vi "Cobra_Front_Panel_Vision_4k.vi"() -> ()   [LabVIEW 2015]
uses:
  <vilib>/vision/Measure.llb/Edge Options.ctl
  <vilib>/vision/Measure.llb/Edge Polarity.ctl
  <vilib>/vision/NI_Vision_Development_Module.lvlib
panel:
  in  "Save Button":bool
  in  "RESET Button":bool
  in  "Process":T1(ring)=enum."Get All Edges"
  in  "Edge Options":T2={"Edge Polarity"=0, "Kernel Size"=3, "Width"=3, "Minimum Edge Strength"=10.0, "Interpolation Type"=enum."Bilinear Fixed", "Data Processing Method"=enum."Average"} {"Edge Polarity" items=["All Edges", "Rising Edges", "Falling Edges"]; "Minimum Edge Strength" format="%.2f"; "Width" step=2; "Kernel Size" step=2}
  out "Line Profile":cluster{"x0":sgl, "dx":sgl, "Pixels Line":sgl[]}(graph)={"x0"=0.0, "dx"=1.0, "Pixels Line"=[]}
  out "Image":T4(plugin-control)
  out "Gradient Information":dbl[](graph)
  in  "Internal Trigger":bool=TRUE
  in  "EXIT":bool
  in  "Line Scan Enable":bool=TRUE
  in  "Line Time Value":u16=90 step=1
  in  "Integration Time Value":u16=100 min=1 max=32767 step=1
  in  "Offset Value":u16=255 max=255 step=1
  in  "Gain Value":u16=187 max=255 step=1
  out "Configuration String Sent":string
  out "Failure":bool
  out "Initialized":bool
  in  "Set":bool
  out "Characters Read":u32
  out "IMAQ Session Out":refnum<k11>
  out "Command Data Read":string
  out "Error Output":errorcluster
  in  "error in (no error)":errorcluster
  # "Suggested Starting Values:\n\nGain: 187\nOffset: 255\nIntegration Time: 90\nLine Time: 100"
  # "Inital Setup and Connection:\n\n  1. Launch NI MAX, select the camera (should be img0).\n  2. Load the supplied *.icd file for the camera.\n  3. Close NI MAX.\n  4. Run this VI and click the \"Set all\" button.\n  5. Stop VI, wait two seconds and run it again to view data"
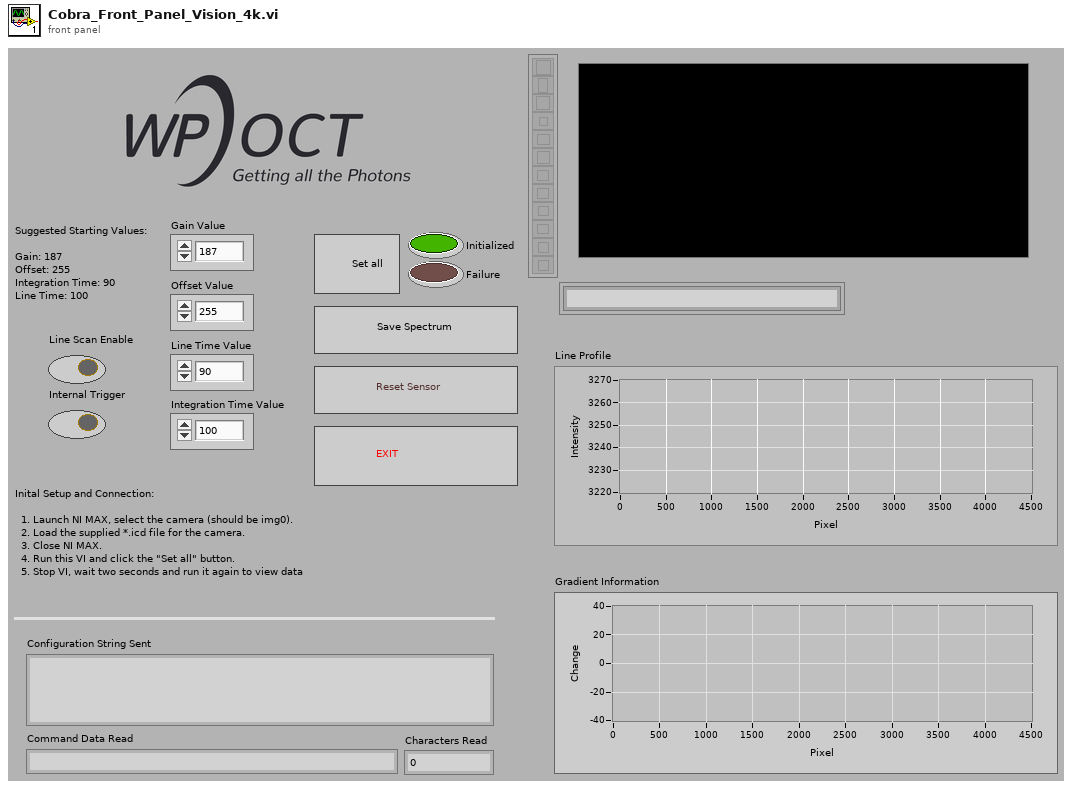
[diagram p1: front panel]
types:
  T1 = enum16{"Get First Edge", "Get First + Last Edge", "Get All Edges", "Get Best Edge"}
  T2 = typedef "Edge Options.ctl" = cluster{"Edge Polarity":T3, "Kernel Size":u32, "Width":u32, "Minimum Edge Strength":sgl, "Interpolation Type":enum32{"Zero Order", "Bilinear", "Quadratic", "Cubic", "Bilinear Fixed"}, "Data Processing Method":enum32{"Average", "Median"}}
  T3 = typedef "Edge Polarity.ctl" = u32
  T4 = typedef "IMAQ Image.ctl" = refnum<image>
  T5 = cluster{"Global Rectangle":i32[], "Contours":cluster{"Contour Type":u32, "ROI Type":u32, "Points":i32[]}[]}
  T6 = typedef "Edge New.ctl" = cluster{"Location (Pixel)":cluster{"X":sgl, "Y":sgl}, "Location (Real-World)":cluster{"X":sgl, "Y":sgl}, "Distance (Pixel)":dbl, "Distance (Real-World)":dbl, "Strength":dbl, "Noise":dbl, "Rising?":bool}
  T7 = typedef "imagedata.ctl" = cluster{"image type":i32, "image depth":i32, "image":u8[], "mask":u8[], "colors":u32[], "Rectangle":cluster{"left":i16, "top":i16, "right":i16, "bottom":i16}}
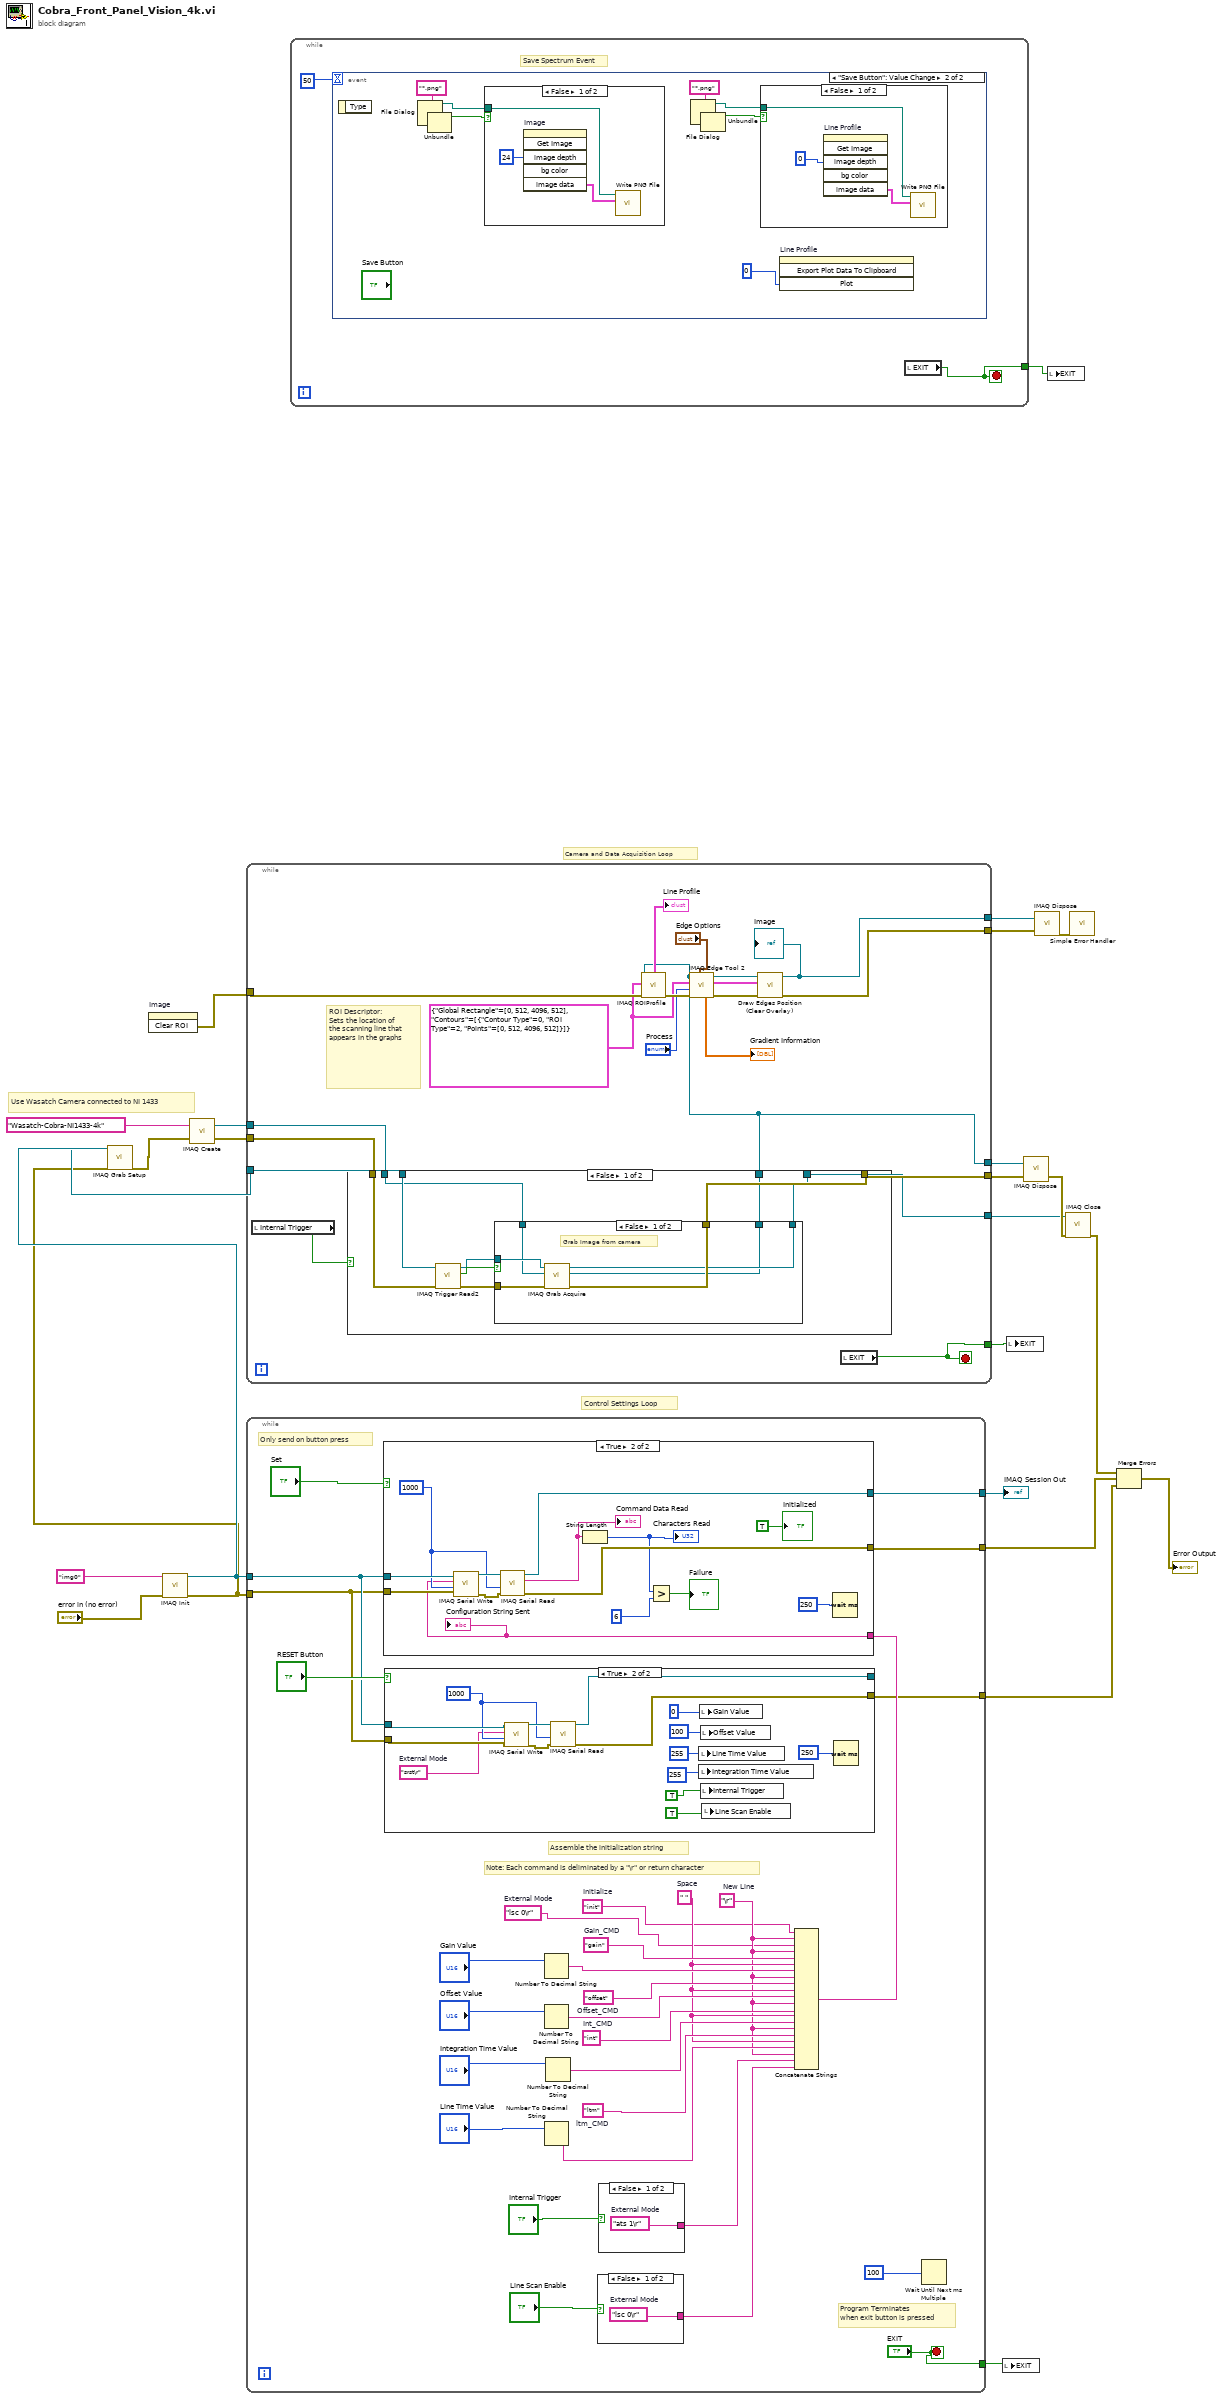
[diagram p0: block diagram]
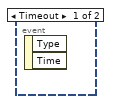
[diagram p2: hidden frame]
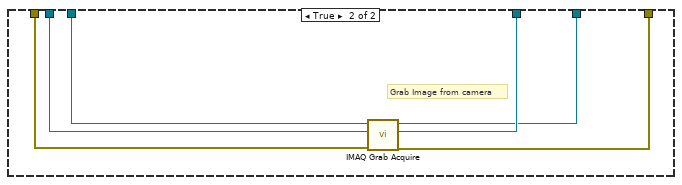
[diagram p6: hidden frame]
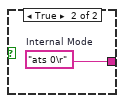
[diagram p8: hidden frame]
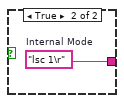
[diagram p10: hidden frame]
diagram:
  # "Use Wasatch Camera connected to NI 1433"
  # "Camera and Data Acquisition Loop"
  # "Control Settings Loop"
  n1 = invoke on="Image" class="ImageControl" method="Clear ROI"() -> (error out=w7:errorcluster)  [unwired: 3 in, 2 out]
  n2 = call <vilib>:"IMAQ Init.vi"("error in (no error)"="error in (no error)", "Interface Name"="img0") -> ("error out"=w21:errorcluster, "IMAQ Session Out"=w23:refnum<k11>)  [unwired: 8 in]
  n3 = call <vilib>:"IMAQ Grab Setup.vi"("error in (no error)"=w21, "IMAQ Session In"=w23) -> ("error out"=w20:errorcluster, "IMAQ Session Out"=w22:refnum<k11>)  [unwired: 8 in]
  n4 = call "IMAQ Create"("Image Name"="Wasatch-Cobra-NI1433-4k", "error in (no error)"=w20) -> ("New Image"=w18:T4, "error out"=w19:errorcluster)  [unwired: 3 in]
  n5 = while {
    tunnel: w23 -> [w29]
    tunnel: w21 -> [w28]
    tunnel: [w55] -> w24
    tunnel: [w54] -> w13
    tunnel: [w27] -> w4
    tunnel: ["EXIT"] -> w3
    stop <- "EXIT" stop-if-true
    w35 = "lsc 0\r"  # External Mode
    w43 = "ltm"  # ltm_CMD
    w42 = "int"  # Int_CMD
    w41 = "offset"  # Offset_CMD
    w40 = "gain"  # Gain_CMD
    w37 = " "  # Space
    w36 = "\r"  # New Line
    w34 = "init"  # Initialize
    # "Program Terminates\nwhen exit button is pressed"
    # "Only send on button press"
    # "Note: Each command is deliminated by a \"\\r\" or return character"
    # "Assemble the initialization string"
    n6 = case shown="True" "RESET Button" {
      tunnel: w29 -> [w57 w67]
      tunnel: w28 -> [w56 w65]
      tunnel: [w57 w72] -> _
      tunnel: [w56 w71] -> w27
      frame False {
      }
      frame True {
        w64 = "srst\r"  # External Mode
        w66 = 1000
        n7 = call <vilib>:"IMAQ Serial Write.vi"("error in (no error)"=w65, "Timeout"=w66, "String to write"=w64, "IMAQ Session In"=w67) -> ("error out"=w68:errorcluster, "IMAQ Session Out"=w69:refnum<k11>)  [unwired: 4 in]
        n8 = call <vilib>:"IMAQ Serial Read.vi"("error in (no error)"=w68, "Timeout"=w66, "IMAQ Session In"=w69) -> ("error out"=w71:errorcluster, "IMAQ Session Out"=w72:refnum<k11>)  [unwired: 3 in, 2 out]
        n9 = local write "Line Time Value"(255) -> ()
        n10 = local write "Integration Time Value"(255) -> ()
        n11 = local write "Gain Value"(0) -> ()
        n12 = local write "Offset Value"(100) -> ()
        n13 = local write "Internal Trigger"(TRUE) -> ()
        n14 = local write "Line Scan Enable"(TRUE) -> ()
        n15 = Wait (ms)(milliseconds to wait=250) -> ()  [unwired: 1 out]
      }
    }
    n16 = Number To Decimal String(number="Gain Value") -> (decimal integer string=w44:string)  [unwired: 1 in]
    n17 = Number To Decimal String(number="Offset Value") -> (decimal integer string=w46:string)  [unwired: 1 in]
    n18 = Number To Decimal String(number="Line Time Value") -> (decimal integer string=w51:string)  [unwired: 1 in]
    n19 = Number To Decimal String(number="Integration Time Value") -> (decimal integer string=w49:string)  [unwired: 1 in]
    n20 = case shown="False" "Line Scan Enable" {
      tunnel: [w91 w92] -> w31
      frame False {
        w91 = "lsc 0\r"  # External Mode
      }
      frame True {
        w92 = "lsc 1\r"  # Internal Mode
      }
    }
    n21 = case shown="False" "Internal Trigger" {
      tunnel: [w73 w74] -> w32
      frame False {
        w73 = "ats 1\r"  # External Mode
      }
      frame True {
        w74 = "ats 0\r"  # Internal Mode
      }
    }
    n22 = Concatenate Strings(w34, w36, w35, w36, w40, w37, w44, w36, w41, w37, w46, w36, w42, w37, w49, w36, w43, w37, w51, w36, w32, w31) -> (w39:string)
    n23 = case shown="True" "Set" {
      tunnel: w29 -> [w76 w84]
      tunnel: w28 -> [w75 w82]
      tunnel: [w76 w90] -> w55
      tunnel: [w75 w89] -> w54
      tunnel: w39 -> [_ w81]
      frame False {
      }
      frame True {
        w83 = 1000
        n24 = call <vilib>:"IMAQ Serial Write.vi"("error in (no error)"=w82, "Timeout"=w83, "String to write"=w81, "IMAQ Session In"=w84) -> ("error out"=w85:errorcluster, "IMAQ Session Out"=w86:refnum<k11>)  [unwired: 4 in]
        n25 = call <vilib>:"IMAQ Serial Read.vi"("error in (no error)"=w85, "Timeout"=w83, "IMAQ Session In"=w86) -> ("error out"=w89:errorcluster, "String Read"=w80:string, "IMAQ Session Out"=w90:refnum<k11>)  [unwired: 3 in, 1 out]
        "Command Data Read" <- w80
        n26 = String Length(string=w80) -> (length=w79:i32)
        "Characters Read" <- w79
        n27 = Greater?(x=w79, y=6) -> (0:→"Failure":bool)
        n28 = Wait (ms)(milliseconds to wait=250) -> ()  [unwired: 1 out]
        "Configuration String Sent" <- w81
        "Initialized" <- TRUE
      }
    }
    n29 = Wait Until Next ms Multiple(millisecond multiple=100) -> ()  [unwired: 1 out]
  }
  "IMAQ Session Out" <- w24
  n30 = while {
    tunnel: w22 -> [w97]
    tunnel: w19 -> [w99]
    tunnel: w18 -> [w98]
    tunnel: [w96] -> w17
    tunnel: [w95] -> w16
    tunnel: [w94] -> w14
    tunnel: w7 -> [w106]
    tunnel: [w105] -> w6
    tunnel: [w102] -> w5
    tunnel: [w101] -> w2
    stop <- w101 stop-if-true
    w93 = T5 {"Global Rectangle"=[0, 512, 4096, 512], "Contours"=[{"Contour Type"=0, "ROI Type"=2, "Points"=[0, 512, 4096, 512]}]} ("NewVal")
    # "ROI Descriptor:\nSets the location of the scanning line that appears in the graphs"
    n31 = local read "Internal Trigger"() -> (w100:bool)
    n32 = case shown="False" w100 {
      tunnel: w99 -> [w119 w135]
      tunnel: w98 -> [w115 w134]
      tunnel: w97 -> [w120 w133]
      tunnel: [w114 w132] -> w96
      tunnel: [w112 w131] -> w95
      tunnel: [w113 w130] -> w94
      frame False {
        n33 = call <vilib>:"IMAQ Trigger Read2.vi"("error in (no error)"=w119, "IMAQ Session In"=w120) -> ("error out"=w118:errorcluster, "Trigger status"=w117:bool, "IMAQ Session Out"=w116:refnum<k11>)  [unwired: 7 in]
        n34 = case shown="False" w117 {
          tunnel: w118 -> [w126 w129]
          tunnel: w116 -> [w125 w128]
          tunnel: w115 -> [w124 w127]
          tunnel: [w123 w129] -> w114
          tunnel: [w122 w128] -> w113
          tunnel: [w121 w127] -> w112
          frame False {
            # "Grab Image from camera"
            n35 = call <vilib>:"IMAQ Grab Acquire.vi"("error in (no error)"=w126, "Image In"=w124, "IMAQ Session In"=w125) -> ("error out"=w123:errorcluster, "Image Out"=w121:T4, "IMAQ Session Out"=w122:refnum<k11>)  [unwired: 5 in, 1 out]
          }
          frame True {
          }
        }
      }
      frame True {
        # "Grab Image from camera"
        n36 = call <vilib>:"IMAQ Grab Acquire.vi"("error in (no error)"=w135, "Image In"=w134, "IMAQ Session In"=w133) -> ("error out"=w132:errorcluster, "Image Out"=w131:T4, "IMAQ Session Out"=w130:refnum<k11>)  [unwired: 5 in, 1 out]
      }
    }
    n37 = call "IMAQ ROIProfile"("error in (no error)"=w106, "ROI Descriptor"=w93, "Image"=w95) -> ("error out"=w111:errorcluster, "ROI Graph"=→"Line Profile":cluster{"x0":sgl, "dx":sgl, "Pixels Line":sgl[]})  [unwired: 4 out]
    n38 = call "IMAQ Edge Tool 2"("Edge Options"="Edge Options", "error in (no error)"=w111, "Process"="Process", "ROI Descriptor"=w93, "Image"=w95) -> ("error out"=w105:errorcluster, "Edge Information"=w108:T6[], "Image (duplicate)"=w109:T4, "Gradient Values"=→"Gradient Information":dbl[])  [unwired: 1 in, 2 out]
    n39 = call "Draw Edges Position (Clear Overlay).vi"("Edge Coordinates"=w108, "Source Image"=w109) -> ("Image Out"=w102:T4)  [unwired: 9 out]
    "Image" <- w102
    n40 = local read "EXIT"() -> (w101:bool)
  }
  n41 = while {
    tunnel: [w137] -> w1
    stop <- w137 stop-if-true
    # "Save Spectrum Event"
    n42 = event shown="[1] \"Save Button\": Value Change" {
      selector: _ -> [_ _]
      dyn-events: _ -> [_ _]
      timeout: 50 -> [_ _]
      event Timeout {
        n43 = event-data() -> ()  [unwired: 1 in, 2 out]
      }
      event "Save Button": Value Change {
        n44 = event-data() -> ()  [unwired: 1 in, 1 out]
        n45 = File Dialog(6:"*.png" ("pattern")) -> (0:w146:errorcluster, 1:w144:bool, 3:w143:path)  [unwired: 6 in, 1 out]
        n46 = Unbundle(w146) -> ()  [unwired: 3 out]
        n47 = case shown="False" w144 {
          tunnel: w143 -> [w152 _]
          frame False {
            n48 = invoke on="Image" class="ImageControl" method="Get Image"("image depth"=24) -> ("image data"=w150:T7)  [unwired: 5 in, 5 out]
            n49 = call <vilib>:"Write PNG File.vi"("image data"=w150, "path to PNG file"=w152) -> ()  [unwired: 8 in, 2 out]
          }
          frame True {
          }
        }
        n50 = File Dialog(6:"*.png" ("pattern")) -> (0:w142:errorcluster, 1:w140:bool, 3:w139:path)  [unwired: 6 in, 1 out]
        n51 = Unbundle(w142) -> ()  [unwired: 3 out]
        n52 = case shown="False" w140 {
          tunnel: w139 -> [w149 _]
          frame False {
            n53 = invoke on="Line Profile" class="WFGraph (strict)" method="Get Image"("image depth"=0) -> ("image data"=w147:T7)  [unwired: 5 in, 5 out]
            n54 = call <vilib>:"Write PNG File.vi"("image data"=w147, "path to PNG file"=w149) -> ()  [unwired: 8 in, 2 out]
          }
          frame True {
          }
        }
        n55 = invoke on="Line Profile" class="WFGraph (strict)" method="Export Plot Data To Clipboard"("Plot"=0 ("image depth")) -> ()  [unwired: 3 in, 4 out]
      }
    }
    n56 = local read "EXIT"() -> (w137:bool)
  }
  n57 = local write "EXIT"(w3) -> ()
  n58 = local write "EXIT"(w2) -> ()
  n59 = call "IMAQ Dispose"("Image"=w16, "error in (no error)"=w17) -> ("error out"=w15:errorcluster)  [unwired: 4 in]
  n60 = call "IMAQ Dispose"("Image"=w5, "error in (no error)"=w6) -> ("error out"=w8:errorcluster)  [unwired: 1 in, 3 out]
  n61 = local write "EXIT"(w1) -> ()
  n62 = call <vilib>:"IMAQ Close.vi"("error in (no error)"=w15, "IMAQ Session In"=w14) -> ("error out"=w10:errorcluster)  [unwired: 9 in]
  n63 = call <vilib>:"Simple Error Handler.vi"("error in (no error)"=w8) -> ()  [unwired: 1 in, 8 out]
  n64 = Merge Errors(w10, w13, w4) -> (→"Error Output":errorcluster)
